vi "Read Components.vi"(8 "error in (no error)":errorcluster, 11 "1553 Board in":refnum<class "1553 Session.lvclass">) -> (0 "error out":errorcluster, 2 "Components":refnum<class "1553 Component.lvclass">[](array[class]), 3 "1553 Board out":refnum<class "1553 Session.lvclass">)   [LabVIEW 2020, in "BCI-1553 API.lvlib" / "1553 Session.lvclass"]
doc: "Read accessor for 1553 Session Components. Depending on the 1553 Session configuration, there may be up to 8 Components in a 1553 Session. When using this accessor and modifying Components, be sure to run the Write Components accessor to update the changes made on the Components."
uses:
  1553 Session.lvclass
  1553 Component/1553 Component.lvclass
  1553 Session.lvclass/1553 Session.ctl
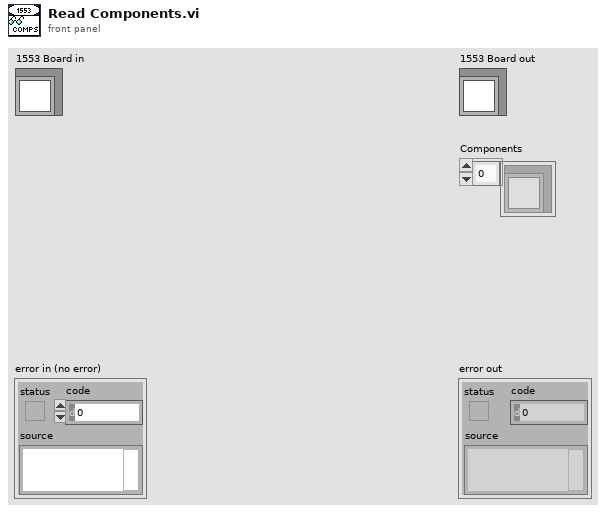
[diagram p1: front panel]
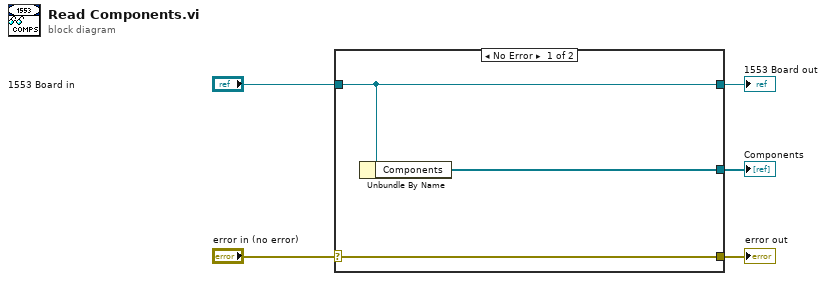
[diagram p0: block diagram]
diagram:
  n1 = case shown="No Error" "error in (no error)" {
    selector: "error in (no error)" -> [w8 w9]
    tunnel: [w8 w9] -> w4
    tunnel: [w7 w10] -> w2
    tunnel: "1553 Board in" -> [w7 w10]
    tunnel: [w6 _] -> w1
    frame No Error {
      n2 = Unbundle By Name(w7) -> ("Components"=w6:refnum<class "1553 Component.lvclass">[])
    }
    frame Error {
    }
  }
  "error out" <- w4
  "1553 Board out" <- w2
  "Components" <- w1
